vi "openAnalysis.vi"(8 "error in (no error)":errorcluster, 10 "ImageAnalyser":refnum<class "ImageAnalyser.lvclass">, 11 "ImageStreamViewer in":refnum<class "ImageStreamViewer.lvclass">) -> (0 "error out":errorcluster, 3 "ImageStreamViewer out":refnum<class "ImageStreamViewer.lvclass">)   [LabVIEW 2009, in "Views.lvlib" / "Camera.lvlib" / "ImageStreamViewer.lvclass"]
uses:
  ImageStreamViewer.lvclass
  Tools/ImageProcessor/ImageAnalyser/ImageAnalyser.lvclass
  ImageStreamViewer.lvclass/ImageStreamViewer.ctl
  Tools/Filing/FileSystem/FileSystem.lvclass
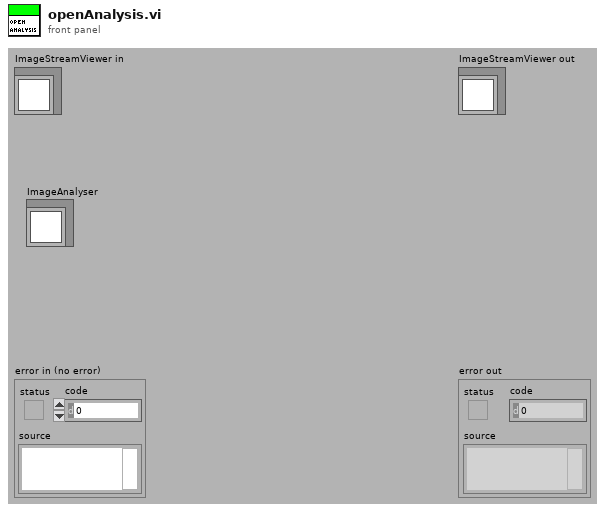
[diagram p1: front panel]
types:
  T1 = enum32{"Invalid", "Standard", "Closed", "Hidden", "Minimized", "Maximized"}
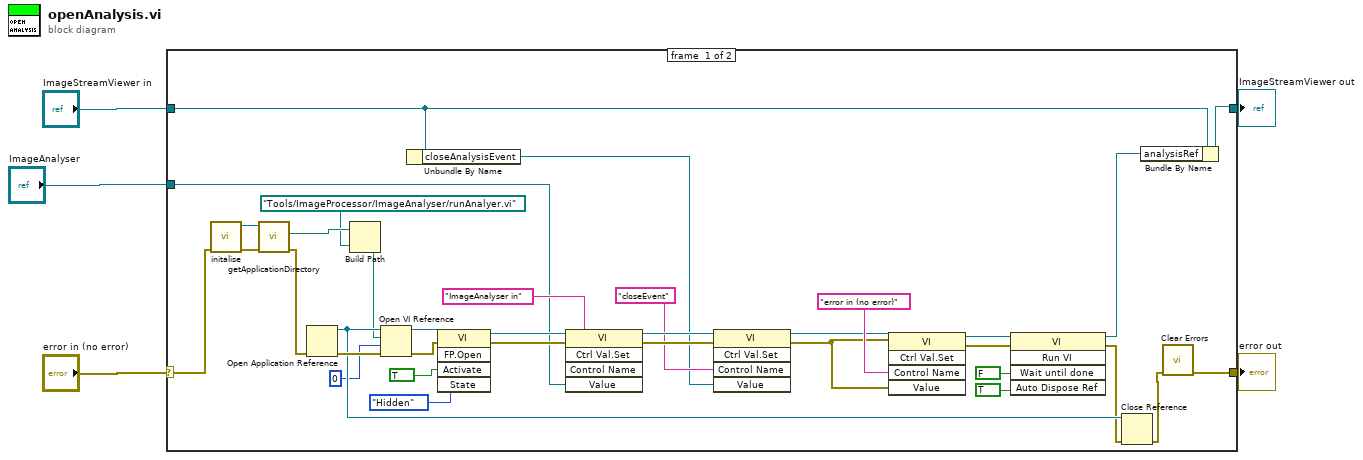
[diagram p0: block diagram]
diagram:
  n1 = case shown="No Error" "error in (no error)" {
    selector: "error in (no error)" -> [w17 w42]
    tunnel: [w9 w42] -> w4
    tunnel: [w6 w41] -> w2
    tunnel: "ImageStreamViewer in" -> [w8 w41]
    tunnel: "ImageAnalyser" -> [w16 _]
    frame #0 {
      n2 = call "initalise.vi"("error in (no error)"=w17) -> ("error out"=w22:errorcluster, "FileSystem out"=w21:refnum<class "FileSystem.lvclass">)  [unwired: 9 in]
      n3 = call-dynamic "getApplicationDirectory.vi"("error in (no error)"=w22, "FileSystem.lvclass in"=w21) -> ("error out"=w20:errorcluster, "ApplicationDirectory"=w24:path)  [unwired: 7 in, 1 out]
      n4 = Open Application Reference(8:w20) -> (0:w37:errorcluster, 3:w35:refnum<vi>)  [unwired: 3 in]
      n5 = Build Path(base path=w24, name or relative path=path "Tools/ImageProcessor/ImageAnalyser/runAnalyer.vi" ("vi path")) -> (appended path=w19:path)
      n6 = Open VI Reference(application reference (local)=w35, vi path=w19, options=0, error in (no error)=w37) -> (vi reference=w31:refnum<vi>, error out=w30:errorcluster)  [unwired: 2 in]
      n7 = Unbundle By Name(w8) -> ("closeAnalysisEvent"=w10:refnum<user-event>)
      n8 = invoke class="VI" method="FP.Open"(reference=w31, error in=w30, "Activate"=TRUE, "State"=T1."Hidden") -> (reference out=w29:refnum<vi>, error out=w28:errorcluster)  [unwired: 1 in, 3 out]
      n9 = invoke class="VI" method="Ctrl Val.Set"(reference=w29, error in=w28, "Control Name"="ImageAnalyser in", "Value"=w16) -> (reference out=w36:refnum<vi>, error out=w13:errorcluster)  [unwired: 1 in, 3 out]
      n10 = invoke class="VI" method="Ctrl Val.Set"(reference=w36, error in=w13, "Control Name"="closeEvent", "Value"=w10) -> (reference out=w14:refnum<vi>, error out=w12:errorcluster)  [unwired: 1 in, 3 out]
      n11 = invoke class="VI" method="Ctrl Val.Set"(reference=w14, error in=w12, "Control Name"="error in (no error)", "Value"=w12) -> (reference out=w33:refnum<vi>, error out=w32:errorcluster)  [unwired: 1 in, 3 out]
      n12 = invoke class="VI" method="Run VI"(reference=w33, error in=w32, "Wait until done"=FALSE, "Auto Dispose Ref"=TRUE) -> (reference out=w7:refnum<vi>, error out=w34:errorcluster)  [unwired: 1 in, 3 out]
      n13 = Close Reference(reference=w35, error in (no error)=w34) -> (error out=w15:errorcluster)
      n14 = Bundle By Name(cluster=w8, "analysisRef"=w7) -> (w6:refnum<class "ImageStreamViewer.lvclass">)
      n15 = call <vilib>:"Clear Errors.vi"("error in (no error)"=w15) -> ("error out"=w9:errorcluster)  [unwired: 6 in]
    }
    frame #1 {
    }
  }
  "error out" <- w4
  "ImageStreamViewer out" <- w2
